vi "Actor Core.vi"(8 "error in":errorcluster, 11 "Linear_Task in":refnum<class "Linear_Task.lvclass">) -> (0 "error out":errorcluster, 3 "Actor out":refnum<class "Actor.lvclass">)   [LabVIEW 2025, in "Linear_Task.lvlib" / "Linear_Task.lvclass"]
doc: "<p>(<strong>Filename</strong>: <span class=\"dnl\">Actor Framework.lvlib:Actor.lvclass:Actor Core.vi</span>)</p>\n<p>Receives messages to the actor, reacts to them, and initiates any error handling that may shut the actor down.</p>\n<p>Descendant classes may override this VI to append parallel tasks for the actor to complete while it handles messages. Overrides use the <a href=\"nihelplauncher://docs/csh?context=lvcore_glang_udclass\">Call Parent Class Method</a> node.</p>"
uses:
  Linear_Task.lvclass
  <vilib>/ActorFramework/Actor/Actor.lvclass
  Linear_Task.lvclass/Linear_Task.ctl
  <vilib>/ActorFramework/Actor/Actor.lvclass/Actor.ctl
  <vilib>/ActorFramework/Message Enqueuer/Message Enqueuer.lvclass/Message Enqueuer.ctl
  Linear_Task Messages/SwitchChart Msg/SwitchChart Msg.lvclass/SwitchChart Msg.ctl
  <vilib>/ActorFramework/Message Enqueuer/Init from Existing Queue.vi
  <vilib>/ActorFramework/Message Enqueuer/Enqueue.vi
  Linear_Task Messages/SwitchChart Msg/SwitchChart Msg.lvclass
  <vilib>/ActorFramework/Message Priority Queue/Priority Enqueue.vi
  <vilib>/ActorFramework/Message Enqueuer/Message Enqueuer.lvclass
  Task_Abstr/Task_Abstr/Task_Abstr.lvclass
panel:
  out "Waveform Graph":waveform(dbl)[](graph)
  out "Waveform Chart":waveform(dbl)[](graph)
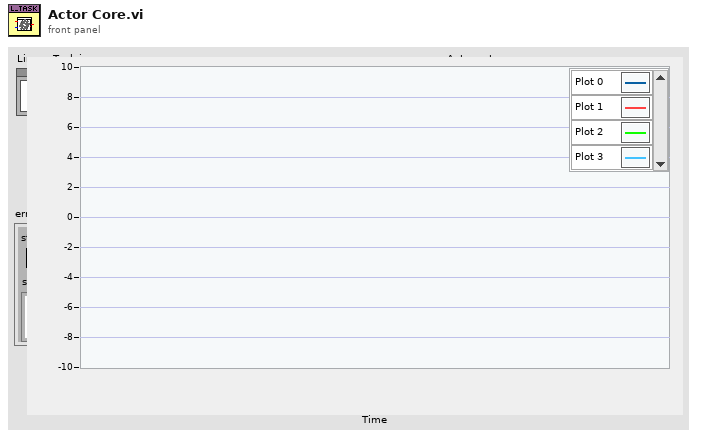
[diagram p1: front panel]
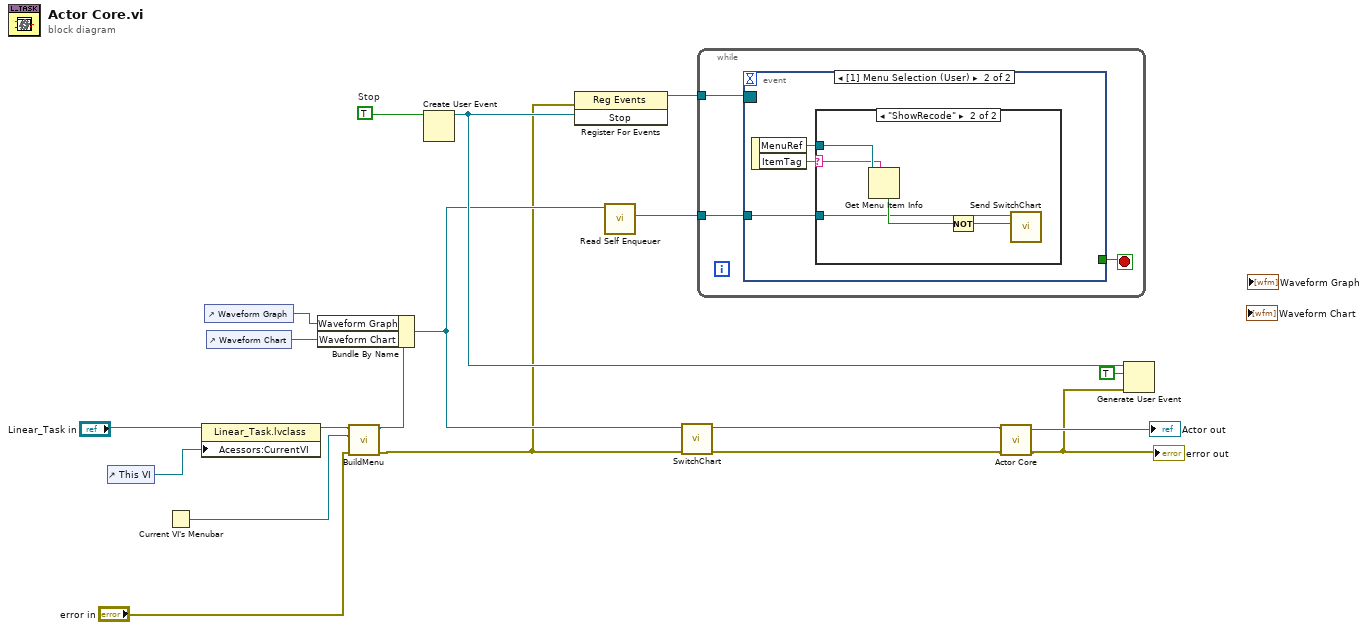
[diagram p0: block diagram]
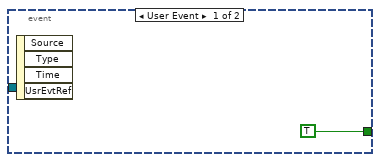
[diagram p2: hidden frame]
diagram:
  w17 = TRUE  # Stop
  n1 = control-ref of="This VI"() -> (w19:refnum<vi>)
  n2 = Current VI's Menubar() -> (w8:refnum<k9>)
  n3 = property class="Linear_Task.lvclass"(reference="Linear_Task in", "Acessors:CurrentVI"=w19) -> (reference out=w10:refnum<class "Linear_Task.lvclass">)  [unwired: 1 in, 1 out]
  n4 = control-ref of="Waveform Graph"() -> (w12:refnum<vi>)
  n5 = control-ref of="Waveform Chart"() -> (w18:refnum<vi>)
  n6 = call "BuildMenu.vi"("error in (no error)"="error in", "menu reference"=w8, "Linear_Task in"=w10) -> ("error out"=w3:errorcluster, "Linear_Task out"=w9:refnum<class "Linear_Task.lvclass">)  [unwired: 7 in]
  n7 = Bundle By Name(cluster=w9, "Waveform Graph"=w12, "Waveform Chart"=w18) -> (w6:refnum<class "Linear_Task.lvclass">)
  n8 = Create User Event(user event datatype=w17) -> (user event=w15:refnum<user-event>)  [unwired: 1 in, 1 out]
  n9 = register-events(error in=w3, w15) -> (reference out=w16:refnum<event-registration>)  [unwired: 1 in, 1 out]
  n10 = call <vilib>:"Read Self Enqueuer.vi"("Actor"=w6) -> ("Self Enqueuer"=w13:refnum<class "Message Enqueuer.lvclass">)  [unwired: 10 in]
  n11 = call "SwitchChart.vi"("error in (no error)"=w3, "Linear_Task in"=w6) -> ("error out"=w4:errorcluster, "Linear_Task out"=w5:refnum<class "Linear_Task.lvclass">)  [unwired: 8 in]
  n12 = while {
    tunnel: w16 -> [w22]
    tunnel: w13 -> [w20]
    stop <- w21 stop-if-true
    n13 = event shown="[1] Menu Selection (User)" {
      selector: w22 -> [_ _]
      dyn-events: _ -> [_ _]
      timeout: _ -> [_ _]
      tunnel: [TRUE _] -> w21
      tunnel: w20 -> [_ w25]
      event User Event {
        n14 = event-data() -> ()  [unwired: 1 in, 4 out]
      }
      event Menu Selection (User) {
        n15 = event-data() -> ("MenuRef"=w24:refnum<k9>, "ItemTag"=w26:string)  [unwired: 1 in]
        n16 = case shown="\"ShowRecode\"" w26 {
          selector: w26 -> [_ w30]
          tunnel: w25 -> [_ w28]
          tunnel: w24 -> [_ w31]
          frame Default {
          }
          frame "ShowRecode" {
            n17 = Get Menu Item Info(7:w30, 11:w31) -> (4:w29:bool)  [unwired: 1 in, 6 out]
            n18 = Not(x=w29) -> (.not. x?=w27:bool)
            n19 = call "Send SwitchChart.vi"("Switch"=w27, "Message Enqueuer"=w28) -> ()  [unwired: 8 in, 2 out]
          }
        }
      }
    }
  }
  n20 = call-parent "Actor Core.vi"("error in"=w4, "Task_Abstr in"=w5) -> ("error out"=w1:errorcluster, "Actor out"=→"Actor out":refnum<class "Actor.lvclass">)  [unwired: 8 in]
  "error out" <- w1
  n21 = Generate User Event(user event=w15, event data cluster=TRUE ("event data"), error in=w1) -> ()  [unwired: 1 in, 2 out]
